vi "Window Blackman-Harris.vi"(1 "Normalize? (False)":bool, 2 "N":i32) -> (0 "window":dbl[](array[numeric]))   [LabVIEW 2020, in "FFTWDLL.lvlib"]
doc: "Blackman-Harris window."
uses:
  FFTWDLL.lvlib
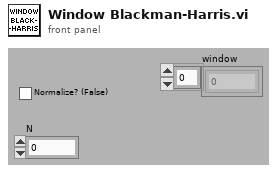
[diagram p1: front panel]
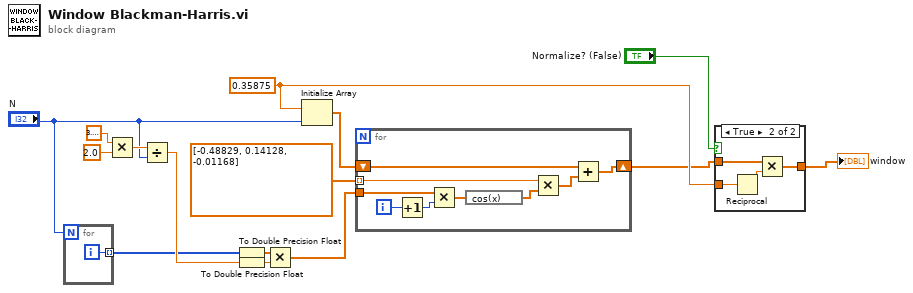
[diagram p0: block diagram]
diagram:
  w2 = 0.35875 ("value")
  n1 = for {
    N: "N" -> [_]
    tunnel: [w16] -> w9 mode=indexing
    i -> [w16]
  }
  n2 = Multiply(x=3.141592653589793, y=2.0) -> (x*y=w13:dbl)
  n3 = Divide(x=w13, y="N") -> (x/y=w10:dbl)
  n4 = To Double Precision Float(number=w9) -> (double precision float=w8:dbl[])
  n5 = To Double Precision Float(number=w10) -> (double precision float=w14:dbl)
  n6 = Multiply(x=w8, y=w14) -> (x*y=w15:dbl[])
  n7 = Initialize Array(w2, "N") -> (w7:dbl[])
  n8 = for {
    shift-right: [w22] -> w1
    shift-left: w7 -> [w21]
    tunnel: dbl[] [-0.48829, 0.14128, -0.01168] -> [w19] mode=indexing
    tunnel: w15 -> [w17]
    i -> [w23]
    n9 = Increment(x=w23) -> (x+1=w24:i32)
    n10 = Multiply(x=w17, y=w24) -> (x*y=w25:dbl[])
    n11 = expression code="cos(x)"(w25) -> (w20:dbl[])
    n12 = Multiply(x=w19, y=w20) -> (x*y=w18:dbl[])
    n13 = Add(x=w21, y=w18) -> (x+y=w22:dbl[])
  }
  n14 = case shown="True" "Normalize? (False)" {
    tunnel: w1 -> [w26 w30]
    tunnel: [w26 w29] -> w4
    tunnel: w2 -> [_ w28]
    frame False {
    }
    frame True {
      n15 = Reciprocal(x=w28) -> (1/x=w27:dbl)
      n16 = Multiply(x=w30, y=w27) -> (x*y=w29:dbl[])
    }
  }
  "window" <- w4
